vi "3.11-Get Critical Critical Points.vi"(0 "Critical Points":T2(array[cluster])) -> (1 "Left Data":T1, 2 "Right Data":T1)   [LabVIEW 2010]
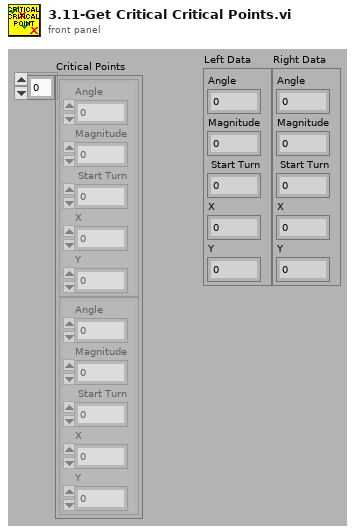
[diagram p1: front panel]
types:
  T1 = cluster{"Angle":dbl, "Magnitude":dbl, " Start Turn":dbl, "X":dbl, "Y":dbl}
  T2 = cluster{"Angle":dbl, "Magnitude":dbl, " Start Turn":dbl, "X":dbl, "Y":dbl}[]
  T3 = cluster{" Angle":dbl, " Magnitude":dbl, " Start Turn":dbl, "X":dbl, "Y":dbl}
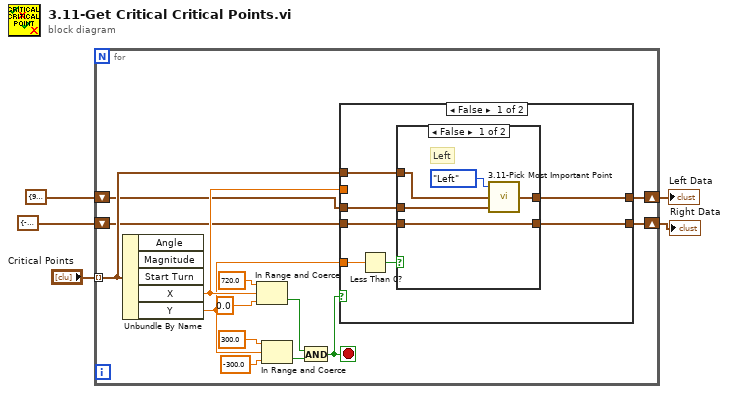
[diagram p0: block diagram]
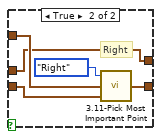
[diagram p2: hidden frame]
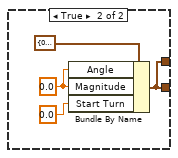
[diagram p3: hidden frame]
diagram:
  n1 = for {
    tunnel: "Critical Points" -> [w8] mode=indexing
    shift-right: [w12] -> w2
    shift-left: T1 {"Angle"=90.0, "Magnitude"=0.0, " Start Turn"=90.0, "X"=-1.0, "Y"=0.0} ("Left Data") -> [w6]
    shift-right: [w11] -> w1
    shift-left: T1 {"Angle"=-90.0, "Magnitude"=0.0, " Start Turn"=-90.0, "X"=-1.0, "Y"=0.0} ("Left Data") -> [w7]
    stop <- w13 stop-if-true
    n2 = Unbundle By Name(w8) -> ("X"=w10:dbl, "Y"=w9:dbl)  [unwired: 3 out]
    n3 = In Range and Coerce(upper limit=720.0, x=w10, lower limit=0.0) -> (In Range?=w14:bool)  [unwired: 1 out]
    n4 = In Range and Coerce(upper limit=300.0, x=w9, lower limit=-300.0) -> (In Range?=w15:bool)  [unwired: 1 out]
    n5 = And(x=w14, y=w15) -> (x .and. y?=w13:bool)
    n6 = case shown="False" w13 {
      tunnel: [w21 w37] -> w12
      tunnel: [w22 w37] -> w11
      tunnel: w10 -> [_ _]
      tunnel: w9 -> [w25 _]
      tunnel: w8 -> [w24 _]
      tunnel: w7 -> [w23 _]
      tunnel: w6 -> [w20 _]
      frame False {
        n7 = Less Than 0?(x=w25) -> (x < 0?=w26:bool)
        n8 = case shown="False" w26 {
          tunnel: w24 -> [w27 w35]
          tunnel: w23 -> [w31 w36]
          tunnel: [w31 w34] -> w22
          tunnel: [w30 w32] -> w21
          tunnel: w20 -> [w28 w32]
          frame False {
            # "Left"
            n9 = call "3.11-Pick Most Important Point.vi"("Old Point"=w28, "New Point"=w27, "Side"=enum16{"Left", "Right"}."Left") -> ("Most Limiting Point"=w30:T3)
          }
          frame True {
            # "Right"
            n10 = call "3.11-Pick Most Important Point.vi"("Old Point"=w36, "New Point"=w35, "Side"=enum16{"Left", "Right"}."Right") -> ("Most Limiting Point"=w34:T3)
          }
        }
      }
      frame True {
        w38 = 0.0 ("Angle")
        n11 = Bundle By Name(cluster=T1 {"Angle"=0.0, "Magnitude"=0.0, " Start Turn"=0.0, "X"=0.0, "Y"=0.0} ("Left Data"), "Angle"=w38, "Magnitude"=w38, "Start Turn"=0.0 ("Angle")) -> (w37:T1)
      }
    }
  }
  "Left Data" <- w2
  "Right Data" <- w1
